vi "Activate Menu Items.vi"(8 "error in (no error)":errorcluster, 9 "State(0)":i32, 10 "Menu Refnum":refnum<k9>, 11 "Menu_Interface in":refnum<class "Menu_Interface.lvclass">) -> (0 "error out":errorcluster, 3 "Menu_Interface out":refnum<class "Menu_Interface.lvclass">)   [LabVIEW 2015, in "Menu_Interface.lvclass"]
uses:
  Menu_Interface.lvclass
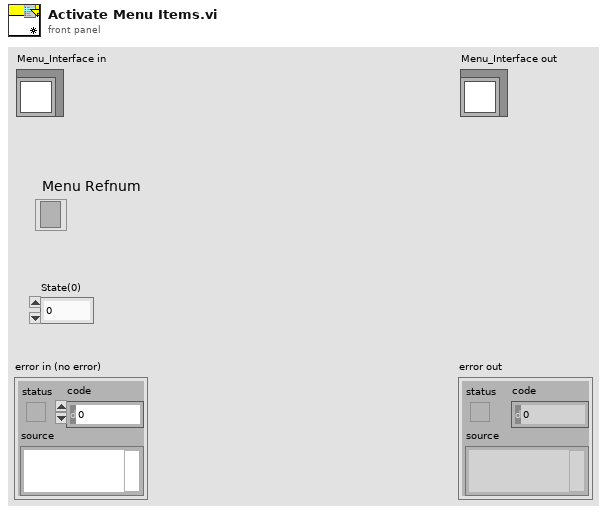
[diagram p1: front panel]
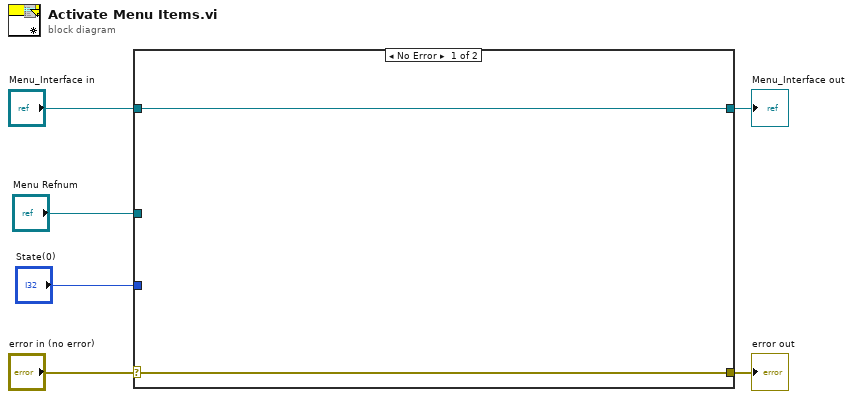
[diagram p0: block diagram]
diagram:
  n1 = case shown="No Error" "error in (no error)" {
    selector: "error in (no error)" -> [w7 w10]
    tunnel: [w7 w10] -> w5
    tunnel: [w8 w9] -> w3
    tunnel: "Menu_Interface in" -> [w8 w9]
    tunnel: "Menu Refnum" -> [_ _]
    tunnel: "State(0)" -> [_ _]
    frame No Error {
    }
    frame Error {
    }
  }
  "error out" <- w5
  "Menu_Interface out" <- w3
